vi "Top-Level.vi"() -> ()   [LabVIEW 2016, in "Webscraper.lvlib"]
uses:
  Webscraper.lvlib
  Type Definitions/Column Type.ctl
  Type Definitions/pyWebscraper Configuration.ctl
  Type Definitions/Row Type.ctl
  Type Definitions/pyWebscraper Test Type.ctl
  Type Definitions/pyWebscraper Image Configuration.ctl
panel:
  in  "Image Configuration":T1={"Images"=[], "Confidence"=0.9} caption="Image Configuration (Only applicable for ratio test)" {"Confidence" min=0.0 max=1.0 format="%.2g"}
  in  "pyWebscraper Test Type":T2
  out "2D Array":string[][](array[string])
  out "standard output":string
  out "element":string
  in  "Row Type":T3
  out "PASS":bool
  in  "pyWebscraper Configuration":T4={"URL"="", "Delay (s)"=10} {"Delay (s)" max=1}
  in  "Column Type":T5
  in  "Python Directory":path caption="(Example: C:\\Users\\chuasy\\AppData\\Local\\Programs\\Python\\Python310)"
  out "error out":errorcluster
  in  "error in (no error)":errorcluster
  # "C:\\Users\\User\\AppData\\Local\\Programs\\Python\\Python312"
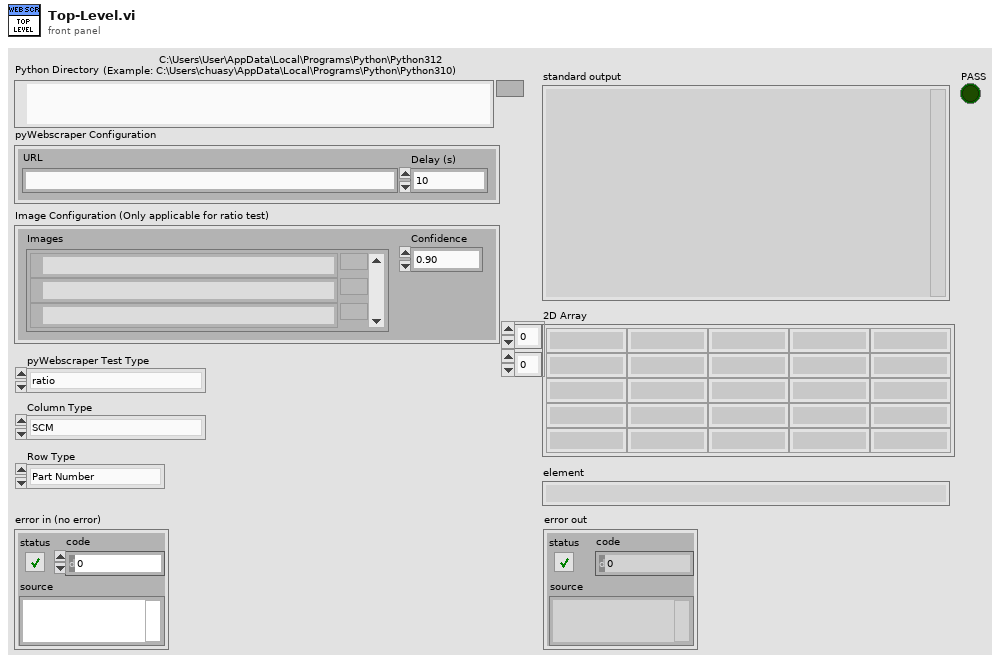
[diagram p1: front panel]
types:
  T1 = typedef "Webscraper.lvlib/pyWebscraper Image Configuration.ctl" = cluster{"Images":path[], "Confidence":dbl}
  T2 = typedef "Webscraper.lvlib/pyWebscraper Test Type.ctl" = enum16{"ratio", "overview", "livepara", "counts", "maxvalue", "alarm_ph2"}
  T3 = typedef "Webscraper.lvlib/Row Type.ctl" = enum16{"Part Number", "Serial Number", "Manufacturing Info", "Manufacturer Name", "Model Revision", "Primary Revision", "Secondary Revision", "LED Status", "Operation", "Current Turn On Time", "Total Turn On Time", "Temperature", "Output Voltage", "Output Current", "Input Voltage", "Input Voltage Type", "Input Power applied", "DC Output ON Cycles", "Output Short Circuit Protection", "Output Over Voltage Protection", "Power Boost", "Over-Temperature Protection", "PS#1 Current High", "PS#1 Temperature High", "PS#1 Input Voltage High", "PS#1 Input Voltage Low", "PS#1 Current Change Threshold", "PS#1 Alarm Enable/Disable", "PS#2 Current High", "PS#2 Temperature High", "PS#2 Input Voltage High", "PS#2 Input Voltage Low", "PS#2 Current Change Threshold", "PS#2 Alarm Enable/Disable", "SCM Temperature High", "SCM Average Temperature Limit", "SCM Alarm Enable/Disable", "Redundancy Alarm Enable/Disable"}
  T4 = typedef "Webscraper.lvlib/pyWebscraper Configuration.ctl" = cluster{"URL":string, "Delay (s)":u32}
  T5 = typedef "Column Type.ctl" = enum16{"SCM", "PS#1", "PS#2", "Name", "Threshold/Status", "Value", "Unit"}
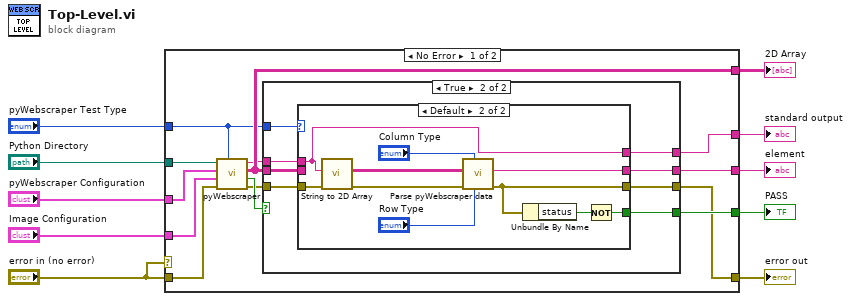
[diagram p0: block diagram]
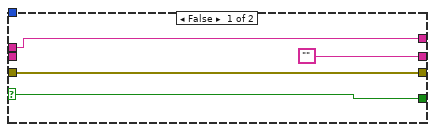
[diagram p2: hidden frame]
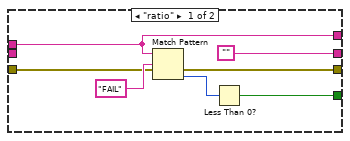
[diagram p3: hidden frame]
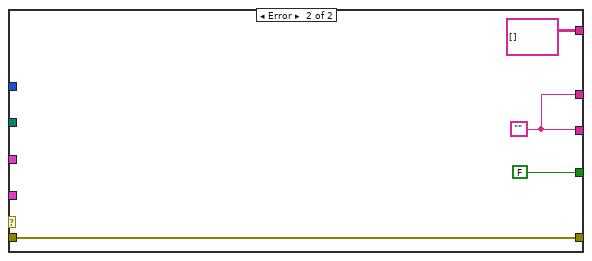
[diagram p4: hidden frame]
diagram:
  n1 = case shown="No Error" "error in (no error)" {
    tunnel: "error in (no error)" -> [w22 w55]
    tunnel: [w16 w55] -> w10
    tunnel: "Python Directory" -> [w23 _]
    tunnel: "pyWebscraper Configuration" -> [w20 _]
    tunnel: [w19 FALSE] -> w7
    tunnel: [w17 w52] -> w6
    tunnel: [w15 string[][] [] ("2D Array")] -> w4
    tunnel: [w12 w52] -> w5
    tunnel: "pyWebscraper Test Type" -> [w14 _]
    tunnel: "Image Configuration" -> [w11 _]
    frame No Error {
      n2 = call "pyWebscraper.vi"("pyWebscraper Test Type"=w14, "error in (no error)"=w22, "Image Configuration"=w11, "pyWebscraper Configuration"=w20, "Python Directory"=w23) -> ("error out"=w18:errorcluster, "PASS"=w21:bool, "2D Array"=w15:string[][], "Output"=w13:string)  [unwired: 3 in]
      n3 = case shown="True" w21 {
        selector: w21 -> [w27 _]
        tunnel: w15 -> [_ w35]
        tunnel: [w27 w34] -> w19
        tunnel: w18 -> [w25 w33]
        tunnel: ["" w32] -> w17
        tunnel: [w25 w31] -> w16
        tunnel: w14 -> [_ w30]
        tunnel: w13 -> [w24 w29]
        tunnel: [w24 w28] -> w12
        frame False {
        }
        frame True {
          n4 = case shown="Default" w30 {
            tunnel: w35 -> [_ _]
            tunnel: [w39 w45] -> w34
            tunnel: w33 -> [w37 w50]
            tunnel: ["" w46] -> w32
            tunnel: [w37 w43] -> w31
            tunnel: w29 -> [w36 w42]
            tunnel: [w36 w42] -> w28
            frame "ratio" {
              n5 = Match Pattern(string=w36, regular expression="FAIL") -> (offset past match=w40:i32)  [unwired: 1 in, 3 out]
              n6 = Less Than 0?(x=w40) -> (x < 0?=w39:bool)
            }
            frame Default {
              n7 = call "String to 2D Array.vi"("error in (no error)"=w50, "String"=w42) -> ("error out"=w49:errorcluster, "2D Array"=w51:string[][])  [unwired: 8 in]
              n8 = call "Parse pyWebscraper data.vi"("Row Type"="Row Type", "Column Type"="Column Type", "error in (no error)"=w49, "2D Array"=w51) -> ("error out"=w43:errorcluster, "element"=w46:string)  [unwired: 6 in]
              n9 = Unbundle By Name(w43) -> ("status"=w44:bool)
              n10 = Not(x=w44) -> (.not. x?=w45:bool)
            }
          }
        }
      }
    }
    frame Error {
      w52 = ""
    }
  }
  "error out" <- w10
  "PASS" <- w7
  "element" <- w6
  "standard output" <- w5
  "2D Array" <- w4
